vi "BuildHWI.vi"(8 "error in (no error)":errorcluster, 10 "Master Device in":refnum<class "Master Device.lvclass">, 11 "Device in":refnum<class "Device.lvclass">) -> (0 "error out":errorcluster, 2 "Master Device out":refnum<class "Master Device.lvclass">, 3 "Device out":refnum<class "Device.lvclass">)   [LabVIEW 2013, in "Device.lvclass"]
doc: "The previous subVI Prune.vi took the \"prepared\" private data and removed unnecessary points. Here in BuildHWI, one should turn the \"prepared\" data into a HWI that can be programmed to the physical device.\n (1) Flatten the data structure and put in normal time order"
uses:
  Device.lvclass
  Master Device/Master Device.lvclass
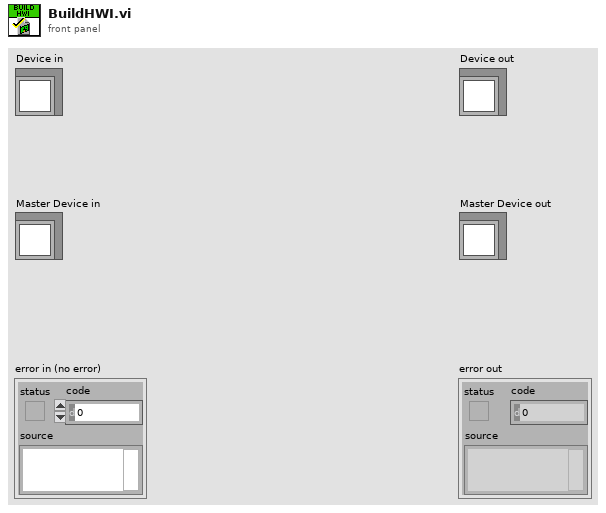
[diagram p1: front panel]
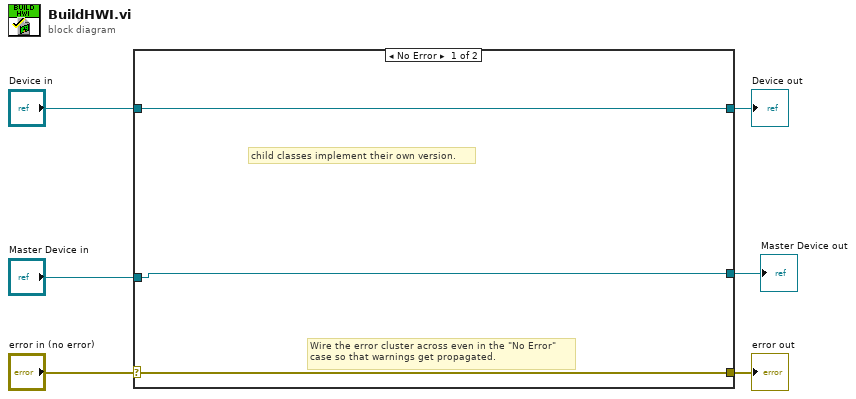
[diagram p0: block diagram]
diagram:
  n1 = case shown="No Error" "error in (no error)" {
    selector: "error in (no error)" -> [w8 w12]
    tunnel: [w8 w12] -> w5
    tunnel: [w9 w11] -> w3
    tunnel: "Device in" -> [w9 w11]
    tunnel: "Master Device in" -> [w7 w10]
    tunnel: [w7 w10] -> w1
    frame No Error {
      # "child classes implement their own version."
      # "Wire the error cluster across even in the \"No Error\"\ncase so that warnings get propagated."
    }
    frame Error {
    }
  }
  "error out" <- w5
  "Device out" <- w3
  "Master Device out" <- w1
